vi "eodrecorder_nearly_complete.vi"() -> ()   [LabVIEW 2012]
uses:
  eodrecorderstates.ctl
  <vilib>/Utility/error.llb/DialogType.ctl
  <vilib>/_DAQmxBase/Internals/DAQmxBase Create Channel (AI-Voltage-Basic).vi
  <vilib>/_DAQmxBase/Internals/DAQmxBase Timing (Sample Clock).vi
  <vilib>/_DAQmxBase/Internals/DAQmxBase Read (Analog 2D DBL NChan NSamp).vi
panel:
  out "WaveformDisplay":T1(array[cluster])
  in  "Polarity":bool=TRUE
  out "Recording Length (sec.)":dbl
  in  "Threshold":sgl
  in  "NumSamptoGrab":i32
  in  "SampleRate":dbl=10000.0
  in  "Channel":tag="Dev1/ai0"
  out "String":string
  out "Tab Control":enum32{"Live Data", "Edit Data", "View Data"}(tab)
  in  "Discard&Continue":bool
  in  "Save&Finish":bool
  in  "Save&Continue":bool
  in  "StartOver":bool
  in  "Tab Control 2":enum32{"Enter Data", "View Data"}(tab)
  out "Time":string
  out "Date":string
  in  "Specimen No.":string
  in  "Locality Code":string
  in  "Recording Temp ûC":string
  in  "Comments":string
  in  "Species":string
  in  "Gain":dbl(knob) scale=0.0..10.0
  in  "Coupling":bool
  in  "Wave Number":u16(slide) scale=0.0..1.0
  out "EodText":string[](array[string])
  out "Polarity":i32[](array[numeric])
  out "Npts":i32[](array[numeric])
  out "Srate":i32[](array[numeric])
  out "ADRange":dbl[](array[numeric])
  in  "WaveNumber":i32(slide) max=4 scale=0.0..5.0
  out "Waveform Graph":dbl[][](graph) caption="Measurement"
  in  "LiveDataMode":bool
  in  "Capture":bool
  in  "Stop":bool
  in  "Open Data":bool
  # "EOD Recorder v. 0.1a"
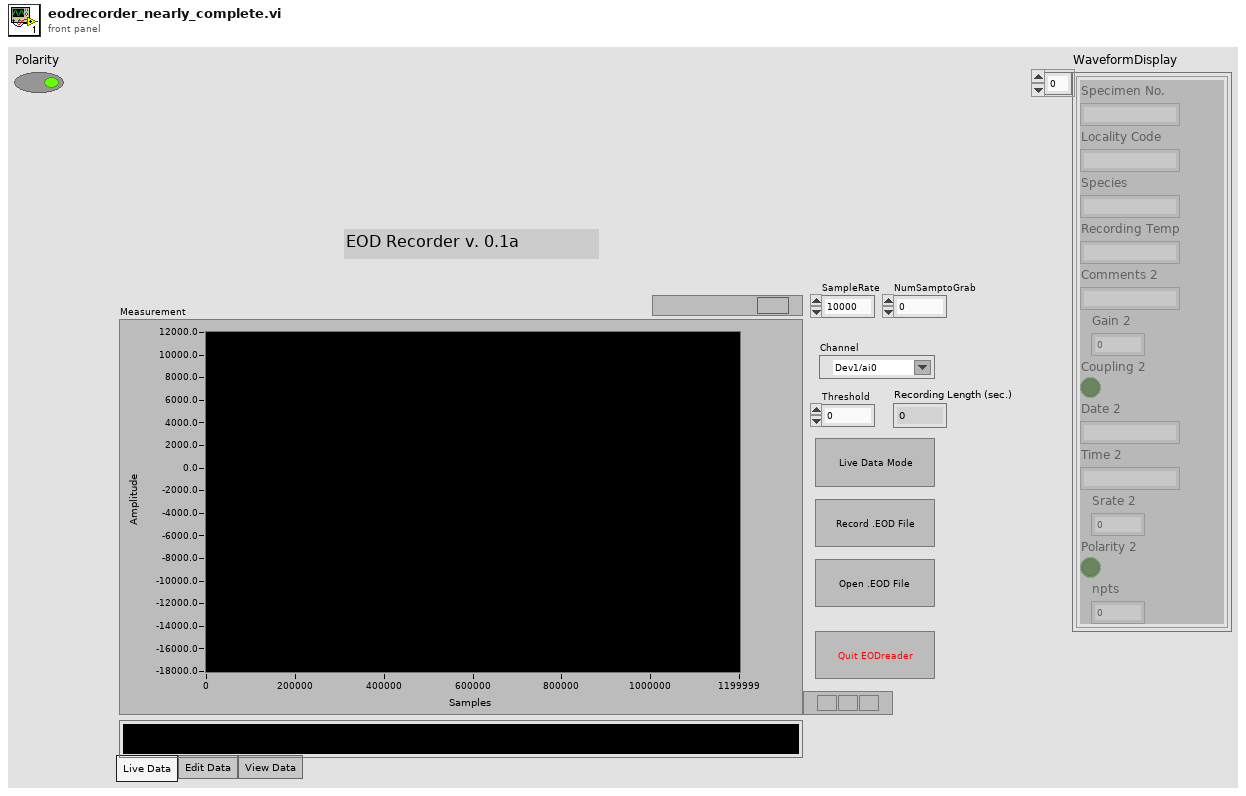
[diagram p1: front panel]
types:
  T1 = cluster{"Specimen No.":string, "Locality Code":string, "Species":string, "Recording Temp":string, "Comments 2":string, "Gain 2":dbl, "Coupling 2":bool, "Date 2":string, "Time 2":string, "Srate 2":dbl, "Polarity 2":bool, "npts":i32}[]
  T2 = cluster{"data":dbl[][], "task ":refnum<k21>, "error ":errorcluster, "Min":dbl, "Max":dbl, "LastGrabbedSrate":dbl, "WaveformData":cluster{"Nchar":i32[], "EodText":string[], "Nbits":i32[], "Nbytes":i32[], "userdata":dbl[][], "Polarity":i32[], "Srate":i32[], "ADRange":dbl[], "Npts":i32[], "Wave":dbl[][]}, "NumberofWavesLoaded":i32, "DescribeWave":cluster{"Specimen 2":string, "Location 2":string, "Species 2":string, "Temp 2":string, "Comments 2":string, "Gain 2":dbl, "Coupling 2":bool, "Date 2":string, "Time 2":string, "Srate 2":dbl, "Polarity 2":bool, "npts":i32}[], "lastgrabbedsamples":i32}
  T3 = typedef "eodrecorderstates.ctl" = enum16{"stop", "initialize", "live data", "capture data", "analyze data", "open data", "display opened data", "write to file"}
  T4 = enum16{"Rising Edge", "Falling Edge", "Above Level", "Below Level", "When Inside Window", "When Outside Window"}
  T5 = enum16{"open", "replace", "create", "open or create", "replace or create", "replace or create with confirmation"}
  T6 = cluster{"Specimen 2":string, "Location 2":string, "Species 2":string, "Temp 2":string, "Comments 2":string, "Gain":dbl, "Coupling":bool, "Date 2":string, "Time 2":string, "Srate":dbl, "Polarity":bool, "npts":i32}
  T7 = enum16{"big-endian, network order", "native, host order", "little-endian"}
  T8 = typedef "DialogType.ctl" = u16
  T9 = cluster{"Nchar":i32[], "EodText":string[], "Nbits":i32[], "Nbytes":i32[], "userdata":dbl[][], "Polarity":i32[], "Srate":i32[], "ADRange":dbl[], "Npts":i32[], "Wave":dbl[][]}
  T10 = cluster{"Specimen 2":string, "Location 2":string, "Species 2":string, "Temp 2":string, "Comments 2":string, "Gain 2":dbl, "Coupling 2":bool, "Date 2":string, "Time 2":string, "Srate 2":dbl, "Polarity 2":bool, "npts":i32}[]
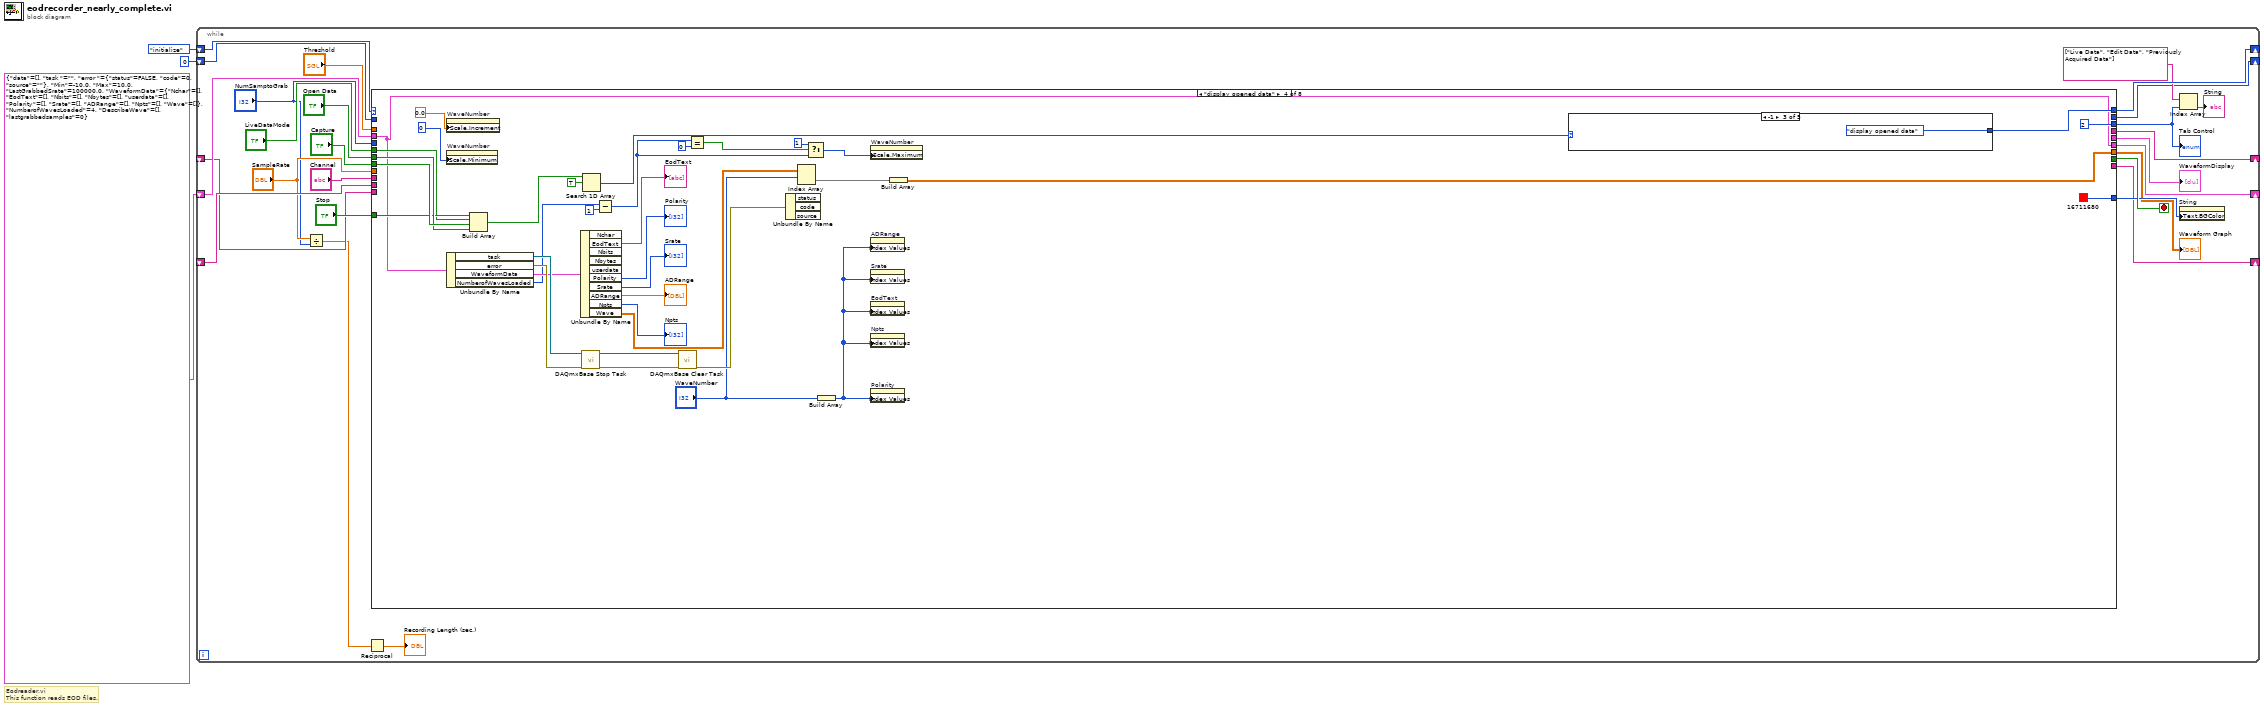
[diagram p0: block diagram]
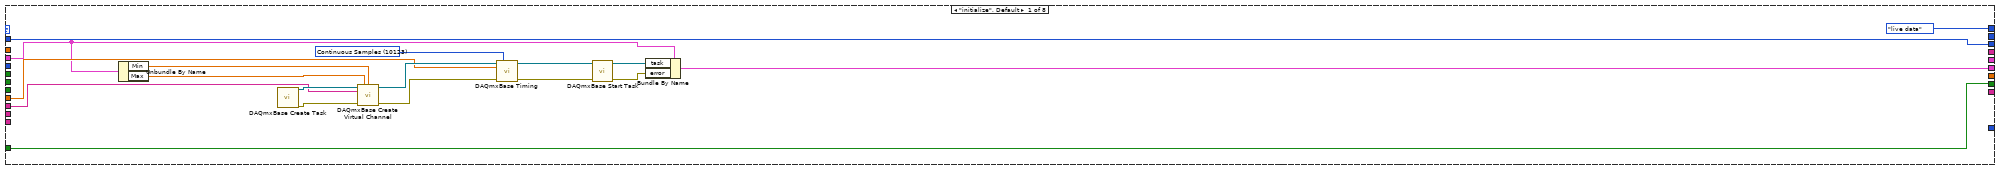
[diagram p2: hidden frame]
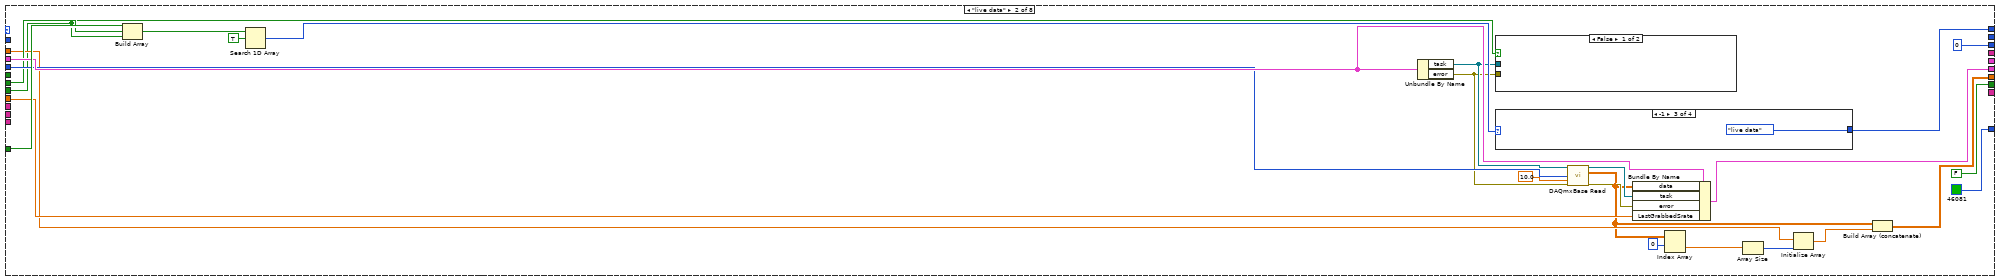
[diagram p3: hidden frame]
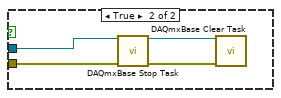
[diagram p4: hidden frame]
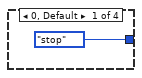
[diagram p5: hidden frame]
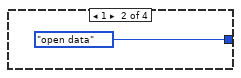
[diagram p6: hidden frame]
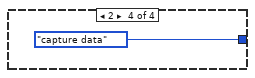
[diagram p7: hidden frame]
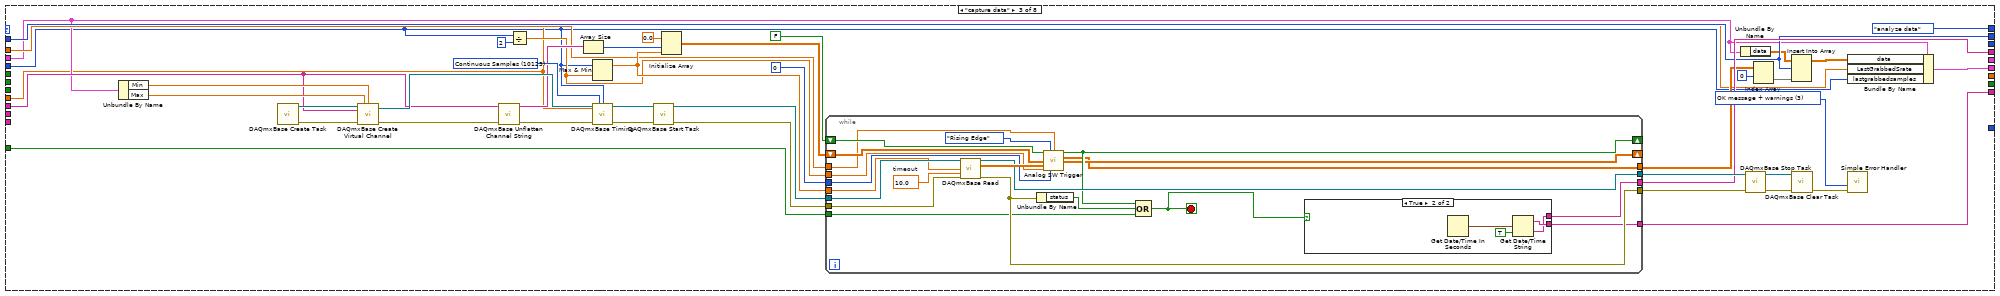
[diagram p8: hidden frame]
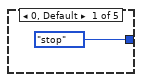
[diagram p10: hidden frame]
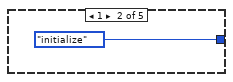
[diagram p11: hidden frame]
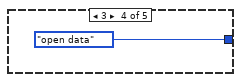
[diagram p12: hidden frame]
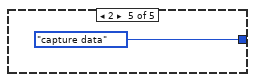
[diagram p13: hidden frame]
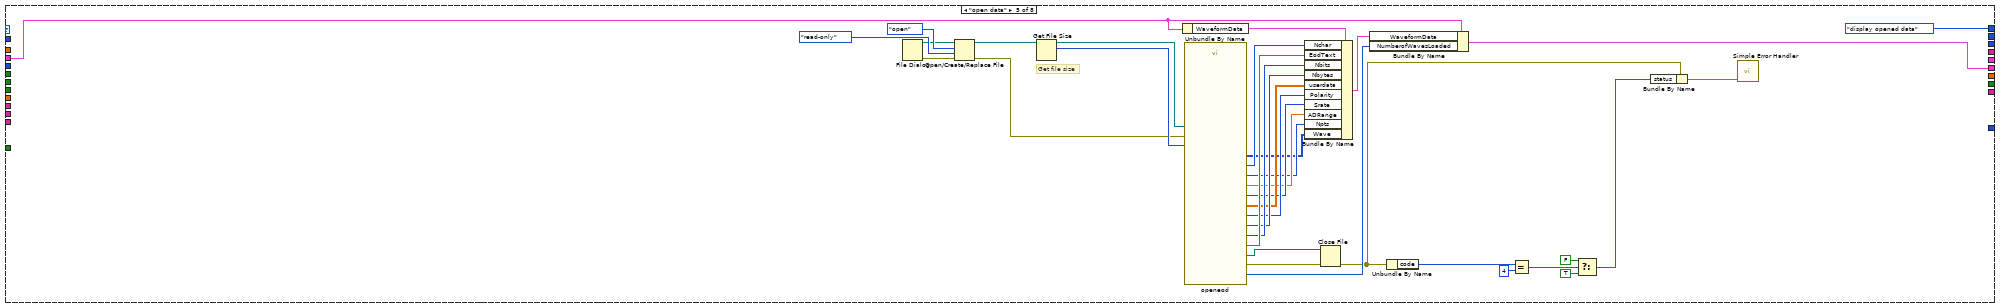
[diagram p14: hidden frame]
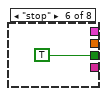
[diagram p15: hidden frame]
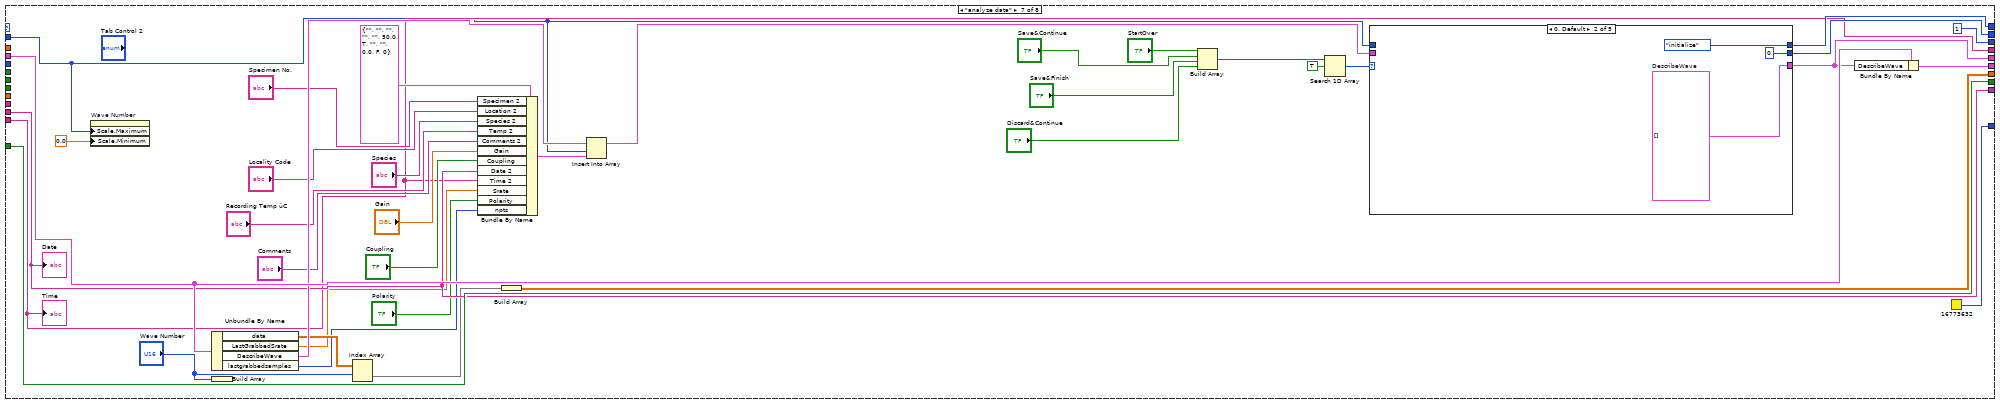
[diagram p16: hidden frame]
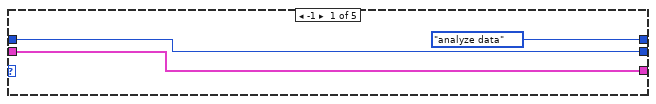
[diagram p17: hidden frame]
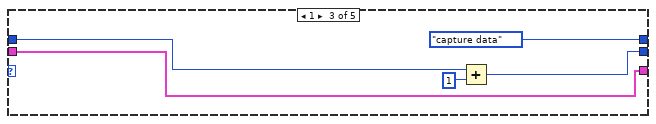
[diagram p18: hidden frame]
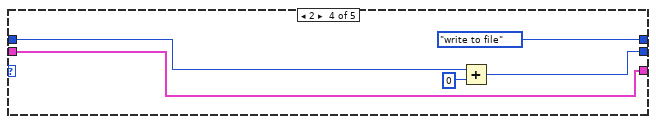
[diagram p19: hidden frame]
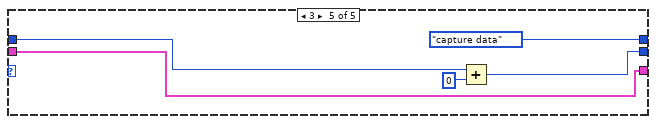
[diagram p20: hidden frame]
diagram:
  # "Eodreader.vi\nThis function reads EOD files."
  n1 = while {
    shift-right: [w29] -> _
    shift-left: eodrecorderstates."initialize" ("Enum") -> [w22]
    shift-right: [w15] -> _
    shift-left: T2 {"data"=[], "task "="", "error "={"status"=FALSE, "code"=0, "source"=""}, "Min"=-10.0, "Max"=10.0, "LastGrabbedSrate"=100000.0, "WaveformData"={"Nchar"=[], "EodText"=[], "Nbits"=[], "Nbytes"=[], "userdata"=[], "Polarity"=[], "Srate"=[], "ADRange"=[], "Npts"=[], "Wave"=[]}, "NumberofWavesLoaded"=4, "DescribeWave"=[], "lastgrabbedsamples"=0} -> [w27]
    shift-right: [w16] -> _
    shift-left: u16 0 -> [w17]
    shift-right: [w12] -> _
    shift-left: _ -> [w10]
    shift-right: [w11] -> _
    shift-left: _ -> [w9]
    stop <- w30 stop-if-true
    n2 = Divide(x="SampleRate", y="NumSamptoGrab") -> (x/y=w5:dbl)
    n3 = Reciprocal(x=w5) -> (1/x=→"Recording Length (sec.)":dbl)
    n4 = case shown="\"display opened data\"" w22 {
      tunnel: [w47 FALSE _ _ _ TRUE w260 _] -> w30
      tunnel: [eodrecorderstates."live data" ("Enum") w73 eodrecorderstates."analyze data" ("Enum") w186 eodrecorderstates."display opened data" ("Enum") _ w259 eodrecorderstates."initialize" ("Enum")] -> w29
      tunnel: "Stop" -> [w47 w72 w100 w180 _ _ w260 _]
      tunnel: w27 -> [w34 w68 w87 w151 w194 _ w250 w313]
      tunnel: "NumSamptoGrab" -> [_ w64 w83 _ _ _ _ _]
      tunnel: "SampleRate" -> [w35 w62 w84 _ _ _ _ _]
      tunnel: "Open Data" -> [_ w63 _ w182 _ _ _ _]
      tunnel: "Capture" -> [_ w60 _ w183 _ _ _ _]
      tunnel: "LiveDataMode" -> [_ _ _ w179 _ _ _ _]
      tunnel: "Threshold" -> [_ w61 w99 _ _ _ _ _]
      tunnel: [w33 0 _ 2 _ _ 1 _] -> w19
      tunnel: [_ u32 46081 _ u32 16711680 _ _ u32 16773632 _] -> w18
      tunnel: w17 -> [w33 _ w89 _ _ _ w230 _]
      tunnel: [_ _ w89 _ _ _ w258 _] -> w16
      tunnel: [w31 w50 w94 w151 w192 _ w249 w313] -> w15
      tunnel: "Channel" -> [w32 _ w95 _ _ _ _ _]
      tunnel: [_ _ _ _ _ _ w247 _] -> w13
      tunnel: [_ _ w93 _ _ _ w237 _] -> w12
      tunnel: [_ _ w92 _ _ _ w236 _] -> w11
      tunnel: w10 -> [_ _ _ _ _ _ w237 _]
      tunnel: w9 -> [_ _ _ _ _ _ w236 _]
      tunnel: [_ w49 _ w152 _ _ w232 _] -> w8
      frame "initialize", Default {
        w42 = 10123 items=["Finite Samples"=10178, "Continuous Samples"=10123] ("sample mode")
        n5 = Unbundle By Name(w34) -> ("Min"=w39:dbl, "Max"=w38:dbl)
        n6 = call <vilib>:"DAQmxBase Create Task.vi"() -> ("task out"=w45:refnum<k21>, "error out"=w46:errorcluster)  [unwired: 5 in, 9 out]
        n7 = call-poly <vilib>:"DAQmxBase Create Virtual Channel.vi"("task in"=w45, "maximum value"=w38, "minimum value"=w39, "physical channels"=w32, "error in"=w46) -> ("task out"=w43:refnum<k21>, "error out"=w44:errorcluster)  [unwired: 4 in, 5 out]
        n8 = call-poly <vilib>:"DAQmxBase Timing.vi"("task/channels in"=w43, "sample mode"=w42, "rate"=w35, "error in"=w44) -> ("task out"=w37:refnum<k21>, "error out"=w36:errorcluster)  [unwired: 3 in, 7 out]
        n9 = call <vilib>:"DAQmxBase Start Task.vi"("task/channels in"=w37, "error in"=w36) -> ("task out"=w41:refnum<k21>, "error out"=w40:errorcluster)  [unwired: 12 out]
        n10 = Bundle By Name(cluster=w34, "task"=w41, "error"=w40) -> (w31:T2)
      }
      frame "live data" {
        n11 = Build Array(w72, w63, w60) -> (w71:bool[])
        n12 = Search 1D Array(1D array=w71, element=TRUE) -> (index of element=w69:i32)  [unwired: 1 in]
        n13 = Unbundle By Name(w68) -> ("task"=w59:refnum<k21>, "error"=w58:errorcluster)
        n14 = case shown="False" w60 {
          tunnel: w59 -> [_ w78]
          tunnel: w58 -> [_ w77]
          frame False {
          }
          frame True {
            n15 = call <vilib>:"DAQmxBase Stop Task.vi"("task/channels in"=w78, "error in"=w77) -> ("task out"=w76:refnum<k21>, "error out"=w75:errorcluster)  [unwired: 12 in]
            n16 = call <vilib>:"DAQmxBase Clear Task.vi"("task in"=w76, "error in"=w75) -> ()  [unwired: 13 in, 1 out]
          }
        }
        n17 = case shown="-1" w69 {
          tunnel: [eodrecorderstates."stop" ("Enum") eodrecorderstates."open data" ("Enum") eodrecorderstates."live data" ("Enum") eodrecorderstates."capture data" ("Enum")] -> w73
          frame 0, Default {
          }
          frame 1 {
          }
          frame -1 {
          }
          frame 2 {
          }
        }
        n18 = call-poly <vilib>:"DAQmxBase Read.vi"("task/channels in"=w59, "number of samples per channel"=w64, "timeout"=10.0, "error in"=w58) -> ("task out"=w67:refnum<k21>, "data"=w53:dbl[][], "error out"=w66:errorcluster)  [unwired: 9 out]
        n19 = Bundle By Name(cluster=w68, "data"=w53, "task"=w67, "error"=w66, "LastGrabbedSrate"=w62) -> (w50:T2)
        n20 = Index Array(array=w53, index (row)=0) -> (element=w55:dbl[])  [unwired: 1 in]
        n21 = Array Size(array=w55) -> (size(s)=w56:i32)
        n22 = Initialize Array(w61, w56) -> (w54:sgl[])
        n23 = Build Array (concatenate)(w53, w54) -> (w49:dbl[][])
      }
      frame "capture data" {
        w105 = T8 3 items=["no dialog", "OK message", "continue or stop message", "OK message + warnings", "continue/stop + warnings"] ("type of dialog (OK msg:1)")
        w125 = 10123 items=["Finite Samples"=10178, "Continuous Samples"=10123] ("sample mode")
        n24 = Unbundle By Name(w87) -> ("Min"=w122:dbl, "Max"=w121:dbl)
        n25 = call <vilib>:"DAQmxBase Create Task.vi"() -> ("task out"=w124:refnum<k21>, "error out"=w123:errorcluster)  [unwired: 14 in]
        n26 = call-poly <vilib>:"DAQmxBase Create Virtual Channel.vi"("task in"=w124, "maximum value"=w121, "minimum value"=w122, "physical channels"=w95, "error in"=w123) -> ("task out"=w120:refnum<k21>, "error out"=w117:errorcluster)  [unwired: 9 in]
        n27 = call "DAQmxBase Unflatten Channel String.vi"("names in"=w95, "error in"=w117) -> ("names out"=w115:string[], "error out"=w116:errorcluster)  [unwired: 12 in]
        n28 = Divide(x=w83, y=2) -> (x/y=w97:dbl)
        n29 = Array Size(array=w115) -> (size(s)=w114:i32)
        n30 = Max & Min(x=w83, y=w97) -> (max(x,y)=w107:dbl)  [unwired: 1 out]
        n31 = call-poly <vilib>:"DAQmxBase Timing.vi"("task/channels in"=w120, "sample mode"=w125, "samples per channel"=w83, "rate"=w84, "error in"=w116) -> ("task out"=w119:refnum<k21>, "error out"=w118:errorcluster)  [unwired: 2 in, 7 out]
        n32 = call <vilib>:"DAQmxBase Start Task.vi"("task/channels in"=w119, "error in"=w118) -> ("task out"=w111:refnum<k21>, "error out"=w112:errorcluster)  [unwired: 12 out]
        n33 = Initialize Array(0.0, w114, w107) -> (w110:dbl[][])
        n34 = while {
          tunnel: [w140] -> w102
          shift-right: [w139] -> _
          shift-left: FALSE ("Trigger Out") -> [w145]
          shift-right: [w133] -> _
          shift-left: w110 -> [w141]
          tunnel: w112 -> [w138]
          tunnel: w111 -> [w137]
          tunnel: w97 -> [w136]
          tunnel: 0 ("Channel Index") -> [w135]
          tunnel: w107 -> [w134]
          tunnel: [w132] -> w91
          tunnel: [w131] -> w101
          tunnel: w100 -> [w130]
          tunnel: w99 -> [w129]
          tunnel: [w127] -> w93
          tunnel: [w126] -> w92
          stop <- w128 stop-if-true
          w146 = 10.0  # timeout
          n35 = call-poly <vilib>:"DAQmxBase Read.vi"("task/channels in"=w137, "number of samples per channel"=w134, "timeout"=w146, "error in"=w138) -> ("task out"=w140:refnum<k21>, "data"=w142:dbl[][], "error out"=w131:errorcluster)  [unwired: 9 in]
          n36 = Unbundle By Name(w131) -> ("status"=w144:bool)
          n37 = call "Analog SW Trigger.vi"("Triggered?"=w145, "Condition"=T4."Rising Edge", "Level"=w129, "Initialized Data Array"=w141, "Input Raw Data"=w142, "Pretrigger Samples"=w136, "Index of Condition Channel"=w135) -> ("Trigger Out"=w139:bool, "Output Data (Scaled)"=w132:dbl[][], "Raw Data Out"=w133:dbl[][])  [unwired: 4 in, 2 out]
          n38 = Compound Arithmetic op=OR(w139, w144, w130) -> (w128:bool)
          n39 = case shown="True" w128 {
            tunnel: [_ w148] -> w127
            tunnel: [_ w147] -> w126
            frame False {
            }
            frame True {
              n40 = Get Date/Time In Seconds() -> (seconds since 1Jan1904=w150:timestamp)
              n41 = Get Date/Time String(seconds (now)=w150, want seconds? (F)=TRUE) -> (date string=w148:string, time string=w147:string)  [unwired: 1 in]
            }
          }
        }
        n42 = Unbundle By Name(w87) -> ("data"=w86:dbl[][])
        n43 = call <vilib>:"DAQmxBase Stop Task.vi"("task/channels in"=w102, "error in"=w101) -> ("task out"=w104:refnum<k21>, "error out"=w103:errorcluster)  [unwired: 12 in]
        n44 = Index Array(array=w91, index (row)=0) -> (element=w85:dbl[])  [unwired: 1 in]
        n45 = Insert Into Array(array=w86, index (row)=w89, new element=w85) -> (w88:dbl[][])  [unwired: 1 in]
        n46 = call <vilib>:"DAQmxBase Clear Task.vi"("task in"=w104, "error in"=w103) -> ("error out"=w106:errorcluster)  [unwired: 13 in]
        n47 = Bundle By Name(cluster=w87, "data"=w88, "LastGrabbedSrate"=w84, "lastgrabbedsamples"=w83) -> (w94:T2)
        n48 = call <vilib>:"Simple Error Handler.vi"("type of dialog (OK msg:1)"=w105, "error in (no error)"=w106) -> ()  [unwired: 3 in, 5 out]
      }
      frame "display opened data" {
        n49 = property on="WaveNumber" class="Slide (strict)"("Scale.Increment"=0.0 ("Scale.Range:Increment")) -> ()  [unwired: 2 in, 2 out]
        n50 = property on="WaveNumber" class="Slide (strict)"("Scale.Minimum"=0) -> ()  [unwired: 2 in, 2 out]
        n51 = Unbundle By Name(w151) -> ("task"=w175:refnum<k21>, "error"=w174:errorcluster, "WaveformData"=w173:T9, "NumberofWavesLoaded"=w153:i32)
        n52 = Build Array(w180, w179, w183, w182) -> (w185:bool[])
        n53 = Unbundle By Name(w173) -> ("EodText"=→"EodText":string[], "Polarity"=→"Polarity":i32[], "Srate"=→"Srate":i32[], "ADRange"=→"ADRange":dbl[], "Npts"=→"Npts":i32[], "Wave"=w165:dbl[][])  [unwired: 4 out]
        n54 = call <vilib>:"DAQmxBase Stop Task.vi"("task/channels in"=w175, "error in"=w174) -> ("task out"=w176:refnum<k21>, "error out"=w177:errorcluster)  [unwired: 12 in]
        n55 = Search 1D Array(1D array=w185, element=TRUE) -> (index of element=w181:i32)  [unwired: 1 in]
        n56 = Subtract(x=w153, y=1) -> (x-y=w157:i32)
        n57 = call <vilib>:"DAQmxBase Clear Task.vi"("task in"=w176, "error in"=w177) -> ("error out"=w178:errorcluster)  [unwired: 13 in]
        n58 = Equal?(x=w157, y=0) -> (x = y?=w158:bool)
        n59 = Unbundle By Name(w178) -> ()  [unwired: 3 out]
        n60 = Index Array(array=w165, index (row)="WaveNumber") -> (element=w163:dbl[])  [unwired: 1 in]
        n61 = Select(t=1, s=w158, f=w157) -> (s? t:f=w155:i32)
        n62 = Build Array("WaveNumber") -> (w167:i32[])
        n63 = property on="WaveNumber" class="Slide (strict)"("Scale.Maximum"=w155) -> ()  [unwired: 2 in, 2 out]
        n64 = property on="ADRange" class="Arr (strict)"("Index Values"=w167) -> ()  [unwired: 2 in, 2 out]
        n65 = property on="Srate" class="Arr (strict)"("Index Values"=w167) -> ()  [unwired: 2 in, 2 out]
        n66 = property on="EodText" class="Arr (strict)"("Index Values"=w167) -> ()  [unwired: 2 in, 2 out]
        n67 = property on="Npts" class="Arr (strict)"("Index Values"=w167) -> ()  [unwired: 2 in, 2 out]
        n68 = property on="Polarity" class="Arr (strict)"("Index Values"=w167) -> ()  [unwired: 2 in, 2 out]
        n69 = Build Array(w163) -> (w152:dbl[][])
        n70 = case shown="-1" w181 {
          tunnel: [eodrecorderstates."stop" ("Enum") eodrecorderstates."initialize" ("Enum") eodrecorderstates."display opened data" ("Enum") eodrecorderstates."open data" ("Enum") eodrecorderstates."capture data" ("Enum")] -> w186
          frame 0, Default {
          }
          frame 1 {
          }
          frame -1 {
          }
          frame 3 {
          }
          frame 2 {
          }
        }
      }
      frame "open data" {
        # "Get file size"
        n71 = File Dialog() -> (0:w221:errorcluster, 3:w222:path)  [unwired: 7 in, 2 out]
        n72 = Open/Create/Replace File(file path (use dialog)=w222, error in=w221, operation (0:open)=T5."open", access (0:read/write)=enum16{"read/write", "read-only", "write-only"}."read-only") -> (refnum out=w210:refnum<file>, error out=w203:errorcluster)  [unwired: 2 in, 1 out]
        n73 = Get File Size(file=w210) -> (refnum out=w209:refnum<file>, size (in bytes)=w208:i64)  [unwired: 1 in, 1 out]
        n74 = Unbundle By Name(w194) -> ("WaveformData"=w220:T9)
        n75 = call "openeod.vi"("Byte Stream File in"=w209, "size (in bytes)"=w208, "error in (no error)"=w203) -> ("Wave"=w193:i16[][], "nchar"=w219:u8[], "polarity"=w215:i8[], "nWavepoints"=w211:u32[], "userdata"=w214:sgl[][], "Numeric"=w206:i32, "nbytes"=w216:i8[], "Byte Stream File out"=w205:refnum<file>, "ADrange"=w212:sgl[], "eodtext"=w218:string[], "srate"=w213:u32[], "nbits"=w217:i8[], "error out"=w204:errorcluster)  [unwired: 4 in]
        n76 = Bundle By Name(cluster=w220, "Nchar"=w219, "EodText"=w218, "Nbits"=w217, "Nbytes"=w216, "userdata"=w214, "Polarity"=w215, "Srate"=w213, "ADRange"=w212, "Npts"=w211, "Wave"=w193) -> (w207:T9)
        n77 = Close File(refnum=w205, error in=w204) -> (error out=w195:errorcluster)  [unwired: 1 out]
        n78 = Bundle By Name(cluster=w194, "WaveformData"=w207, "NumberofWavesLoaded"=w206) -> (w192:T2)
        n79 = Unbundle By Name(w195) -> ("code"=w202:i32)
        n80 = Equal?(x=w202, y=4) -> (x = y?=w200:bool)
        n81 = Select(t=FALSE, s=w200, f=TRUE) -> (s? t:f=w197:bool)
        n82 = Bundle By Name(cluster=w195, "status"=w197) -> (w196:errorcluster)
        n83 = call <vilib>:"Simple Error Handler.vi"("error in (no error)"=w196) -> ()  [unwired: 4 in, 5 out]
      }
      frame "stop" {
      }
      frame "analyze data" {
        n84 = property on="Wave Number" class="Slide (strict)"("Scale.Maximum"=w230, "Scale.Minimum"=0.0 ("Scale.Range:Minimum")) -> ()  [unwired: 2 in, 2 out]
        n85 = Unbundle By Name(w250) -> ("data"=w235:dbl[][], "LastGrabbedSrate"=w229:dbl, "DescribeWave"=w248:T10, "lastgrabbedsamples"=w227:i32)
        n86 = Build Array("Wave Number") -> ()  [unwired: 1 out]
        n87 = Index Array(array=w235, index (row)="Wave Number") -> (element=w233:dbl[])  [unwired: 1 in]
        n88 = Bundle By Name(cluster=T6 {"Specimen 2"="", "Location 2"="", "Species 2"="", "Temp 2"="", "Comments 2"="", "Gain"=50.0, "Coupling"=TRUE, "Date 2"="", "Time 2"="", "Srate"=0.0, "Polarity"=FALSE, "npts"=0} ("WaveformDescribe 2"), "Specimen 2"="Specimen No.", "Location 2"="Locality Code", "Species 2"="Species", "Temp 2"="Recording Temp ûC", "Comments 2"="Comments", "Gain"="Gain", "Coupling"="Coupling", "Date 2"=w237, "Time 2"=w236, "Srate"=w229, "Polarity"="Polarity", "npts"=w227) -> (w238:T6)
        n89 = Build Array(w233) -> (w232:dbl[][])
        n90 = Insert Into Array(array=w248, index=w230, new element=w238) -> (w252:T10)
        n91 = Build Array("StartOver", "Save&Continue", "Save&Finish", "Discard&Continue") -> (w261:bool[])
        n92 = Search 1D Array(1D array=w261, element=TRUE) -> (index of element=w253:i32)  [unwired: 1 in]
        n93 = case shown="0, Default" w253 {
          tunnel: [w265 0 w273 w278 w283] -> w258
          tunnel: w230 -> [w265 _ w272 w277 w282]
          tunnel: [eodrecorderstates."analyze data" ("Enum") eodrecorderstates."initialize" ("Enum") eodrecorderstates."capture data" ("Enum") eodrecorderstates."write to file" ("Enum") eodrecorderstates."capture data" ("Enum")] -> w259
          tunnel: [w264 w267 w270 w275 w280] -> w247
          tunnel: w252 -> [w264 _ w270 w275 w280]
          frame -1 {
          }
          frame 0, Default {
            w267 = T10 []  # DescribeWave
          }
          frame 1 {
            n94 = Add(x=w272, y=1) -> (x+y=w273:i32)
          }
          frame 2 {
            n95 = Add(x=w277, y=0) -> (x+y=w278:i32)
          }
          frame 3 {
            n96 = Add(x=w282, y=0) -> (x+y=w283:i32)
          }
        }
        n97 = Bundle By Name(cluster=w250, "DescribeWave"=w247) -> (w249:T2)
        "Time" <- w236
        "Date" <- w237
      }
      frame "write to file" {
        # "version\nnchar\nwave_text (terminate with null char?)\nnbits\nnbytes\ndata_polarity\nuser_data\ns_rate\nad_range\nnpts\nwave"
        n98 = Unbundle By Name(w313) -> ("data"=w311:dbl[][], "DescribeWave"=w312:T10)  [unwired: 7 out]
        n99 = for {
          tunnel: w312 -> [w362] mode=indexing
          tunnel: w311 -> [w326] mode=indexing
          tunnel: [w361] -> w286 mode=indexing
          tunnel: [w339] -> w294 mode=indexing
          tunnel: [w337] -> w295 mode=indexing
          tunnel: [w336] -> w296 mode=indexing
          tunnel: [w335] -> w293 mode=indexing
          tunnel: [w334] -> w292 mode=indexing
          tunnel: [w331] -> w291 mode=indexing
          tunnel: [w330] -> w290 mode=indexing
          tunnel: [w328] -> w289 mode=indexing
          tunnel: [w327] -> w288 mode=indexing
          tunnel: [w324] -> w287 mode=indexing
          w327 = "65536"  # ADRange
          w330 = "0 0 0 0 0 0"  # UserData
          w334 = "2"  # Nbytes
          w335 = "16"  # Nbits
          w336 = "1"  # Version
          n100 = Unbundle By Name(w362) -> ("Specimen 2"=w353:string, "Location 2"=w352:string, "Species 2"=w351:string, "Temp 2"=w350:string, "Comments 2"=w349:string, "Gain 2"=w348:dbl, "Coupling 2"=w345:bool, "Date 2"=w342:string, "Time 2"=w340:string, "Srate 2"=w329:dbl, "Polarity 2"=w332:bool)  [unwired: 1 out]
          n101 = Array Size(array=w326) -> (size(s)=w325:i32)
          n102 = Number To Decimal String(number=w326) -> (decimal integer string=w361:string[])  [unwired: 1 in]
          n103 = Boolean To (0,1)(Boolean=w345) -> (0, 1=w346:i16)
          n104 = Number To Decimal String(number=w325) -> (decimal integer string=w324:string)  [unwired: 1 in]
          n105 = Number To Decimal String(number=w348) -> (decimal integer string=w347:string)  [unwired: 1 in]
          n106 = Number To Decimal String(number=w346) -> (decimal integer string=w344:string)  [unwired: 1 in]
          n107 = Concatenate Strings(" Date= " ("string"), w342, " Time= " ("string"), w340, "Specimen=" ("string"), w353, " Location= " ("string"), w352, " Species= " ("string"), w351, " Temp= " ("string"), w350, "Gain= " ("string"), w347, " Coupling= " ("string"), w344, " Comments= " ("string"), w349) -> (w339:string)
          n108 = String Length(string=w339) -> (length=w338:i32)
          n109 = Boolean To (0,1)(Boolean=w332) -> (0, 1=w333:i16)
          n110 = Number To Decimal String(number=w338) -> (decimal integer string=w337:string)  [unwired: 1 in]
          n111 = Number To Decimal String(number=w333) -> (decimal integer string=w331:string)  [unwired: 1 in]
          n112 = Number To Decimal String(number=w329) -> (decimal integer string=w328:string)  [unwired: 1 in]
        }
        n113 = Build Array(w296, w295, w294, w293, w292, w291, w290, w289, w288, w287) -> (w297:string[][])
        n114 = Build Array(w286) -> (w285:string[][][])
        n115 = File Dialog(7:"Enter Filename" ("prompt"), 9:"TestFile.EOD" ("default name")) -> (0:w303:errorcluster, 3:w309:path)  [unwired: 5 in, 2 out]
        n116 = Open/Create/Replace File(file path (use dialog)=w309, error in=w303, operation (0:open)=T5."open or create", access (0:read/write)=enum16{"read/write", "read-only", "write-only"}."write-only") -> (refnum out=w305:refnum<file>, error out=w304:errorcluster)  [unwired: 2 in, 1 out]
        n117 = Transpose 2D Array(2D array=w297) -> (transposed array=w298:string[][])
        n118 = for {
          tunnel: T7."native, host order" ("byte order (0:big-endian, network order)") -> [w323]
          tunnel: w305 -> [w322]
          tunnel: w304 -> [w321]
          tunnel: [w319] -> w300
          tunnel: [w318] -> w299
          tunnel: w298 -> [w320] mode=indexing
          tunnel: w285 -> [w315] mode=indexing
          n119 = Write to Binary File(file (use dialog)=w322, data=w320, error in=w321, 9:w323) -> (refnum out=w317:refnum<file>, error out=w316:errorcluster)  [unwired: 2 in, 1 out]
          n120 = Write to Binary File(file (use dialog)=w317, data=w315, error in=w316) -> (refnum out=w319:refnum<file>, error out=w318:errorcluster)  [unwired: 3 in, 1 out]
        }
        n121 = Close File(refnum=w300, error in=w299) -> (error out=w302:errorcluster)  [unwired: 1 out]
        n122 = call <vilib>:"Simple Error Handler.vi"("error in (no error)"=w302) -> ()  [unwired: 4 in, 5 out]
      }
    }
    "Waveform Graph" <- w8
    "Tab Control" <- w19
    "WaveformDisplay" <- w13
    n123 = Index Array(array=string[] ["Live Data", "Edit Data", "Previously Acquired Data"], index=w19) -> (element=→"String":string)
    n124 = property on="String" class="Str"("Text.BGColor"=w18) -> ()  [unwired: 2 in, 2 out]
  }
